vi "Set Comms stop notifier.vi"(10 "Comms stop":refnum<notifier>, 11 "SCADA Communications in":refnum<class "SCADA Communications.lvclass">) -> (3 "SCADA Communications out":refnum<class "SCADA Communications.lvclass">)   [LabVIEW 2015, in "SCADA Communcations Actor.lvlib" / "SCADA Communications.lvclass"]
uses:
  SCADA Communications.lvclass
  SCADA Communications.lvclass/SCADA Communications.ctl
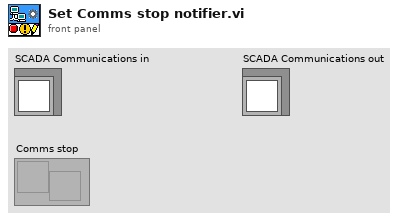
[diagram p1: front panel]
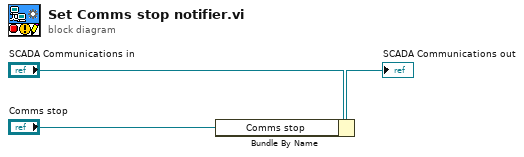
[diagram p0: block diagram]
diagram:
  n1 = Bundle By Name(cluster="SCADA Communications in", "Comms stop"="Comms stop") -> (→"SCADA Communications out":refnum<class "SCADA Communications.lvclass">)
